vi "Ack needed.vi"(11 "Publish JSON in":refnum<class "Publish JSON.lvclass">) -> (2 "Ack needed?":bool, 3 "Publish JSON out":refnum<class "Publish JSON.lvclass">)   [LabVIEW 2020, in "wamplv.lvlib" / "Publish JSON.lvclass"]
uses:
  Publish JSON.lvclass
  Publish JSON.lvclass/Publish JSON.ctl
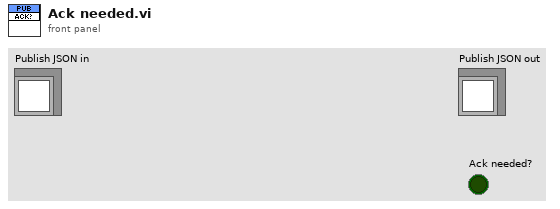
[diagram p1: front panel]
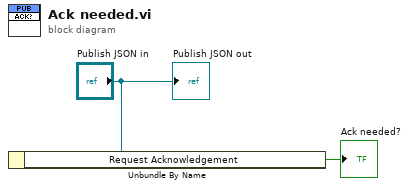
[diagram p0: block diagram]
diagram:
  n1 = Unbundle By Name("Publish JSON in") -> ("Request Acknowledgement"=→"Ack needed?":bool)
  "Publish JSON out" <- "Publish JSON in"
